vi "myBodePlot.vi"(3 "swp_data":dbl[][](array[numeric]), 4 "可用pico数":u16, 5 "幅值单位":u8(ring) items=["dB", "abs"], 8 "响应选项":u8=2, 9 "注入选项":u8=2, 11 "freqs, meas, coups":i32[][](array[numeric])) -> (0 "Pha":cluster{dbl[], dbl[]}[](graph), 1 "Mag":cluster{dbl[], dbl[]}[](graph))   [LabVIEW 2024]
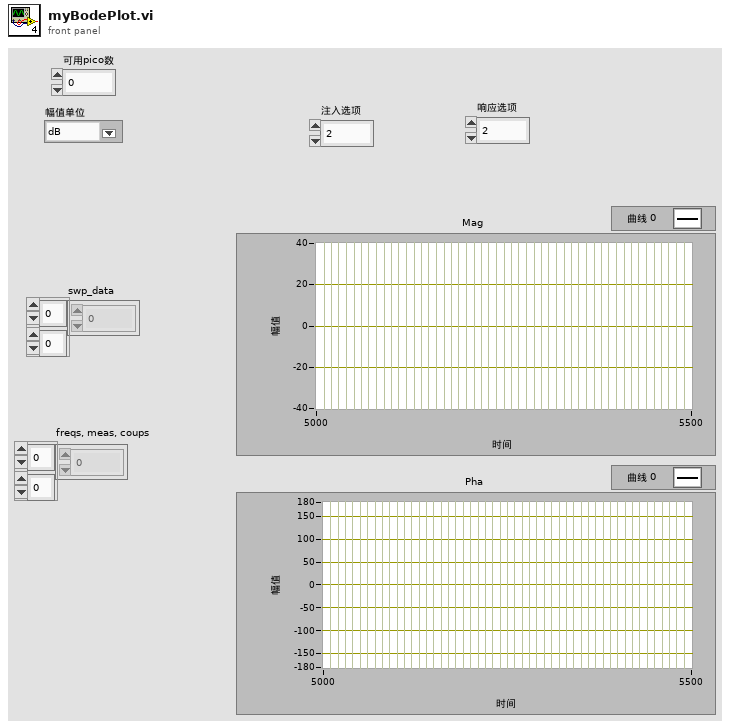
[diagram p1: front panel]
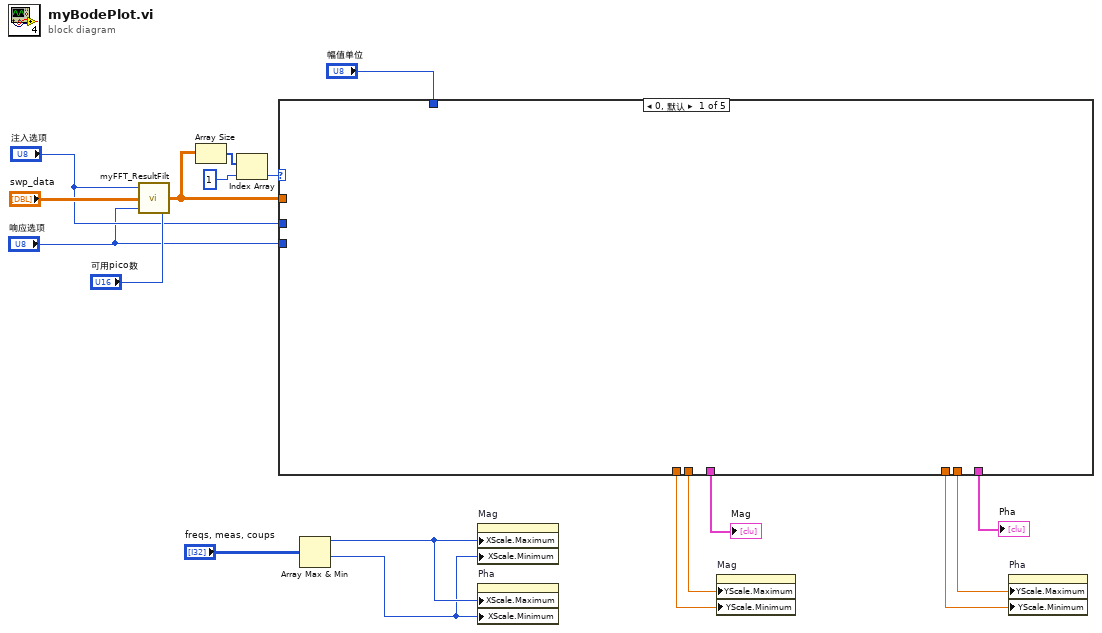
[diagram p0: block diagram]
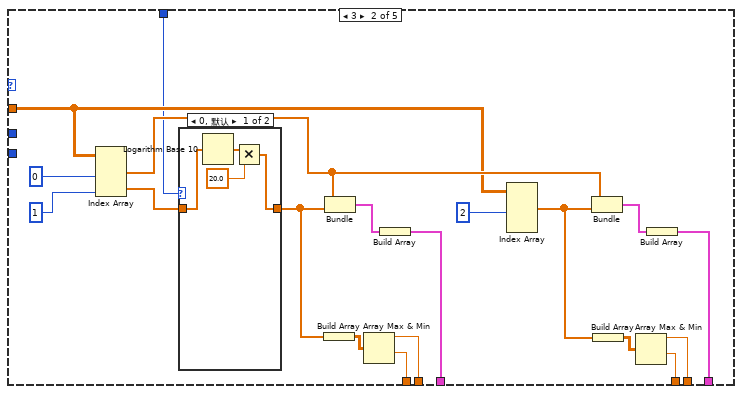
[diagram p2: hidden frame]
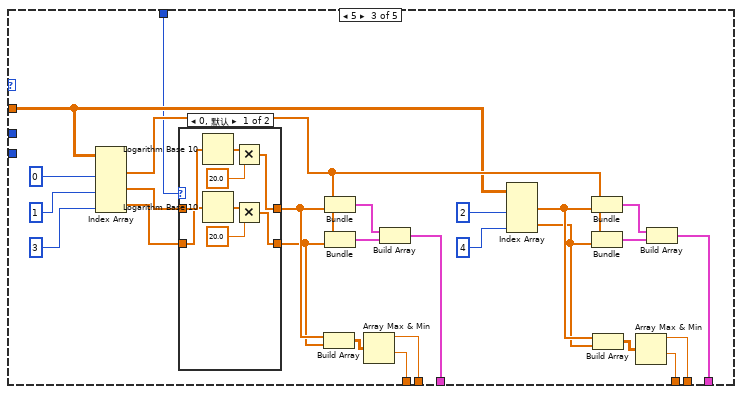
[diagram p4: hidden frame]
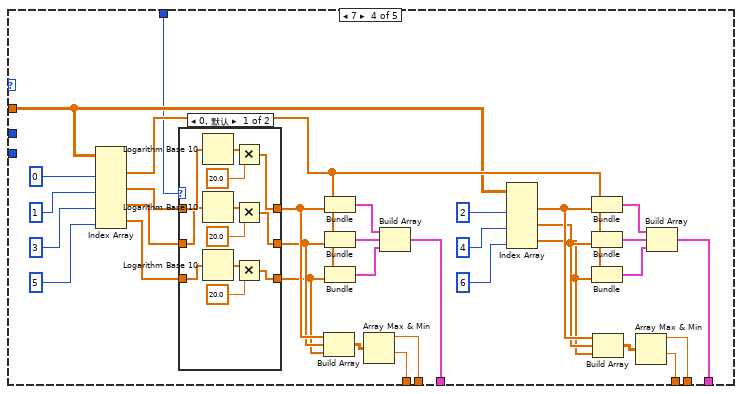
[diagram p6: hidden frame]
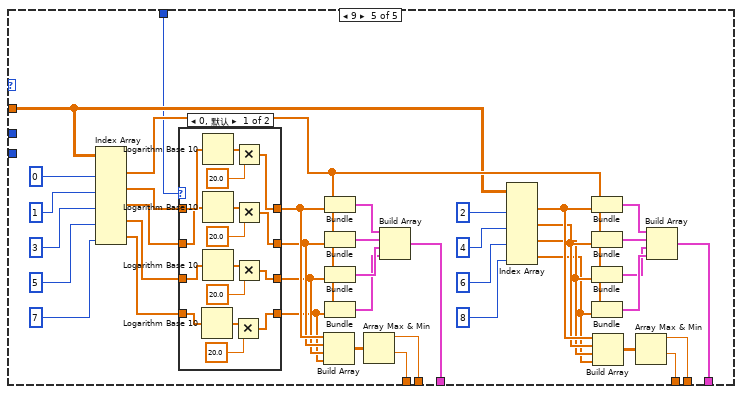
[diagram p8: hidden frame]
diagram:
  n1 = call "myFFT_ResultFilt.vi"("可用PICO数"="可用pico数", "响应选项"="响应选项", "写表结果输入"="swp_data", "注入选项"="注入选项") -> ("写表结果输出"=w2:dbl[][])  [unwired: 1 in]
  n2 = Array Size(array=w2) -> (size(s)=w13:i32[])
  n3 = Index Array(array=w13, index=1 ("索引")) -> (element=w11:i32)
  n4 = case shown="0, 默认" w11 {
    tunnel: "注入选项" -> [_ _ _ _ _]
    tunnel: "响应选项" -> [_ _ _ _ _]
    tunnel: "幅值单位" -> [_ w21 w49 w89 w141]
    tunnel: [_ w28 w56 w96 w148] -> w7
    tunnel: [_ w27 w55 w95 w147] -> w6
    tunnel: [_ w26 w54 w94 w146] -> w5
    tunnel: [_ w25 w53 w93 w145] -> w4
    tunnel: [_ w24 w52 w92 w144] -> w3
    tunnel: w2 -> [_ w23 w51 w91 w143]
    tunnel: [_ w22 w50 w90 w142] -> w1
    frame 0, Default {
    }
    frame 3 {
      n5 = Index Array(array=w23, index (col) #1=0, index (col) #2=1) -> (element #1=w29:dbl[], element #2=w19:dbl[])  [unwired: 2 in]
      n6 = case shown="0, 默认" w21 {
        tunnel: [w39 w42] -> w30
        tunnel: w19 -> [w38 w42]
        frame 0, Default {
          n7 = Logarithm Base 10(1:w38) -> (0:w41:dbl[])
          n8 = Multiply(x=w41, y=20.0) -> (x*y=w39:dbl[])
        }
        frame 1 {
        }
      }
      n9 = Build Array(w30) -> (w33:dbl[][])
      n10 = Bundle("写表结果输出"=w29, "写表结果输出"=w30) -> (w34:cluster{"写表结果输出":dbl[], "写表结果输出":dbl[]})  [unwired: 1 in]
      n11 = Array Max & Min(array=w33) -> (max value=w26:dbl, min value=w25:dbl)  [unwired: 2 out]
      n12 = Build Array(w34) -> (w22:cluster{"写表结果输出":dbl[], "写表结果输出":dbl[]}[])
      n13 = Index Array(array=w23, index (col) #1=2) -> (element #1=w32:dbl[])  [unwired: 3 in, 1 out]
      n14 = Bundle("写表结果输出"=w29, "写表结果输出"=w32) -> (w35:cluster{"写表结果输出":dbl[], "写表结果输出":dbl[]})  [unwired: 1 in]
      n15 = Build Array(w32) -> (w31:dbl[][])
      n16 = Array Max & Min(array=w31) -> (max value=w27:dbl, min value=w28:dbl)  [unwired: 2 out]
      n17 = Build Array(w35) -> (w24:cluster{"写表结果输出":dbl[], "写表结果输出":dbl[]}[])
    }
    frame 5 {
      n18 = Index Array(array=w51, index (col) #1=0, index (col) #2=1, index (col) #3=3) -> (element #1=w57:dbl[], element #2=w46:dbl[], element #3=w45:dbl[])  [unwired: 3 in]
      n19 = case shown="0, 默认" w49 {
        tunnel: [w74 w78] -> w59
        tunnel: w46 -> [w73 w78]
        tunnel: w45 -> [w70 w77]
        tunnel: [w69 w77] -> w58
        frame 0, Default {
          n20 = Logarithm Base 10(1:w73) -> (0:w76:dbl[])
          n21 = Logarithm Base 10(1:w70) -> (0:w71:dbl[])
          n22 = Multiply(x=w76, y=20.0) -> (x*y=w74:dbl[])
          n23 = Multiply(x=w71, y=20.0) -> (x*y=w69:dbl[])
        }
        frame 1 {
        }
      }
      n24 = Build Array(w59, w58) -> (w62:dbl[][])
      n25 = Bundle("写表结果输出"=w57, "写表结果输出"=w59) -> (w63:cluster{"写表结果输出":dbl[], "写表结果输出":dbl[]})  [unwired: 1 in]
      n26 = Bundle("写表结果输出"=w57, "写表结果输出"=w58) -> (w64:cluster{"写表结果输出":dbl[], "写表结果输出":dbl[]})  [unwired: 1 in]
      n27 = Array Max & Min(array=w62) -> (max value=w54:dbl, min value=w53:dbl)  [unwired: 2 out]
      n28 = Build Array(w63, w64) -> (w50:cluster{"写表结果输出":dbl[], "写表结果输出":dbl[]}[])
      n29 = Index Array(array=w51, index (col) #1=2, index (col) #2=4) -> (element #1=w61:dbl[], element #2=w44:dbl[])  [unwired: 2 in]
      n30 = Bundle("写表结果输出"=w57, "写表结果输出"=w61) -> (w66:cluster{"写表结果输出":dbl[], "写表结果输出":dbl[]})  [unwired: 1 in]
      n31 = Bundle("写表结果输出"=w57, "写表结果输出"=w44) -> (w65:cluster{"写表结果输出":dbl[], "写表结果输出":dbl[]})  [unwired: 1 in]
      n32 = Build Array(w61, w44) -> (w60:dbl[][])
      n33 = Array Max & Min(array=w60) -> (max value=w55:dbl, min value=w56:dbl)  [unwired: 2 out]
      n34 = Build Array(w66, w65) -> (w52:cluster{"写表结果输出":dbl[], "写表结果输出":dbl[]}[])
    }
    frame 7 {
      n35 = Index Array(array=w91, index (col) #1=0, index (col) #2=1, index (col) #3=3, index (col) #4=5) -> (element #1=w97:dbl[], element #2=w85:dbl[], element #3=w84:dbl[], element #4=w83:dbl[])  [unwired: 4 in]
      n36 = case shown="0, 默认" w89 {
        tunnel: [w121 w126] -> w100
        tunnel: w85 -> [w120 w126]
        tunnel: w84 -> [w115 w125]
        tunnel: w83 -> [w113 w124]
        tunnel: [w114 w125] -> w99
        tunnel: [w112 w124] -> w98
        frame 0, Default {
          n37 = Logarithm Base 10(1:w120) -> (0:w123:dbl[])
          n38 = Logarithm Base 10(1:w115) -> (0:w118:dbl[])
          n39 = Logarithm Base 10(1:w113) -> (0:w116:dbl[])
          n40 = Multiply(x=w123, y=20.0) -> (x*y=w121:dbl[])
          n41 = Multiply(x=w118, y=20.0) -> (x*y=w114:dbl[])
          n42 = Multiply(x=w116, y=20.0) -> (x*y=w112:dbl[])
        }
        frame 1 {
        }
      }
      n43 = Build Array(w100, w99, w98) -> (w103:dbl[][])
      n44 = Bundle("写表结果输出"=w97, "写表结果输出"=w100) -> (w104:cluster{"写表结果输出":dbl[], "写表结果输出":dbl[]})  [unwired: 1 in]
      n45 = Bundle("写表结果输出"=w97, "写表结果输出"=w99) -> (w105:cluster{"写表结果输出":dbl[], "写表结果输出":dbl[]})  [unwired: 1 in]
      n46 = Bundle("写表结果输出"=w97, "写表结果输出"=w98) -> (w106:cluster{"写表结果输出":dbl[], "写表结果输出":dbl[]})  [unwired: 1 in]
      n47 = Array Max & Min(array=w103) -> (max value=w94:dbl, min value=w93:dbl)  [unwired: 2 out]
      n48 = Build Array(w104, w105, w106) -> (w90:cluster{"写表结果输出":dbl[], "写表结果输出":dbl[]}[])
      n49 = Index Array(array=w91, index (col) #1=2, index (col) #2=4, index (col) #3=6) -> (element #1=w102:dbl[], element #2=w82:dbl[], element #3=w81:dbl[])  [unwired: 3 in]
      n50 = Bundle("写表结果输出"=w97, "写表结果输出"=w102) -> (w109:cluster{"写表结果输出":dbl[], "写表结果输出":dbl[]})  [unwired: 1 in]
      n51 = Bundle("写表结果输出"=w97, "写表结果输出"=w82) -> (w108:cluster{"写表结果输出":dbl[], "写表结果输出":dbl[]})  [unwired: 1 in]
      n52 = Bundle("写表结果输出"=w97, "写表结果输出"=w81) -> (w107:cluster{"写表结果输出":dbl[], "写表结果输出":dbl[]})  [unwired: 1 in]
      n53 = Build Array(w102, w82, w81) -> (w101:dbl[][])
      n54 = Array Max & Min(array=w101) -> (max value=w95:dbl, min value=w96:dbl)  [unwired: 2 out]
      n55 = Build Array(w109, w108, w107) -> (w92:cluster{"写表结果输出":dbl[], "写表结果输出":dbl[]}[])
    }
    frame 9 {
      n56 = Index Array(array=w143, index (col) #1=0, index (col) #2=1, index (col) #3=3, index (col) #4=5, index (col) #5=7) -> (element #1=w149:dbl[], element #2=w136:dbl[], element #3=w135:dbl[], element #4=w134:dbl[], element #5=w133:dbl[])  [unwired: 5 in]
      n57 = case shown="0, 默认" w141 {
        tunnel: [w180 w186] -> w153
        tunnel: w136 -> [w179 w186]
        tunnel: w135 -> [w174 w185]
        tunnel: w134 -> [w172 w184]
        tunnel: w133 -> [w168 w183]
        tunnel: [w173 w185] -> w152
        tunnel: [w171 w184] -> w151
        tunnel: [w167 w183] -> w150
        frame 0, Default {
          n58 = Logarithm Base 10(1:w168) -> (0:w170:dbl[])
          n59 = Logarithm Base 10(1:w179) -> (0:w182:dbl[])
          n60 = Logarithm Base 10(1:w174) -> (0:w177:dbl[])
          n61 = Logarithm Base 10(1:w172) -> (0:w175:dbl[])
          n62 = Multiply(x=w170, y=20.0) -> (x*y=w167:dbl[])
          n63 = Multiply(x=w182, y=20.0) -> (x*y=w180:dbl[])
          n64 = Multiply(x=w177, y=20.0) -> (x*y=w173:dbl[])
          n65 = Multiply(x=w175, y=20.0) -> (x*y=w171:dbl[])
        }
        frame 1 {
        }
      }
      n66 = Build Array(w153, w152, w151, w150) -> (w156:dbl[][])
      n67 = Bundle("写表结果输出"=w149, "写表结果输出"=w153) -> (w157:cluster{"写表结果输出":dbl[], "写表结果输出":dbl[]})  [unwired: 1 in]
      n68 = Bundle("写表结果输出"=w149, "写表结果输出"=w152) -> (w158:cluster{"写表结果输出":dbl[], "写表结果输出":dbl[]})  [unwired: 1 in]
      n69 = Bundle("写表结果输出"=w149, "写表结果输出"=w151) -> (w160:cluster{"写表结果输出":dbl[], "写表结果输出":dbl[]})  [unwired: 1 in]
      n70 = Bundle("写表结果输出"=w149, "写表结果输出"=w150) -> (w159:cluster{"写表结果输出":dbl[], "写表结果输出":dbl[]})  [unwired: 1 in]
      n71 = Array Max & Min(array=w156) -> (max value=w146:dbl, min value=w145:dbl)  [unwired: 2 out]
      n72 = Build Array(w157, w158, w160, w159) -> (w142:cluster{"写表结果输出":dbl[], "写表结果输出":dbl[]}[])
      n73 = Index Array(array=w143, index (col) #1=2, index (col) #2=4, index (col) #3=6, index (col) #4=8) -> (element #1=w155:dbl[], element #2=w132:dbl[], element #3=w131:dbl[], element #4=w127:dbl[])  [unwired: 4 in]
      n74 = Bundle("写表结果输出"=w149, "写表结果输出"=w155) -> (w164:cluster{"写表结果输出":dbl[], "写表结果输出":dbl[]})  [unwired: 1 in]
      n75 = Bundle("写表结果输出"=w149, "写表结果输出"=w132) -> (w163:cluster{"写表结果输出":dbl[], "写表结果输出":dbl[]})  [unwired: 1 in]
      n76 = Bundle("写表结果输出"=w149, "写表结果输出"=w131) -> (w161:cluster{"写表结果输出":dbl[], "写表结果输出":dbl[]})  [unwired: 1 in]
      n77 = Bundle("写表结果输出"=w149, "写表结果输出"=w127) -> (w162:cluster{"写表结果输出":dbl[], "写表结果输出":dbl[]})  [unwired: 1 in]
      n78 = Build Array(w155, w132, w131, w127) -> (w154:dbl[][])
      n79 = Array Max & Min(array=w154) -> (max value=w147:dbl, min value=w148:dbl)  [unwired: 2 out]
      n80 = Build Array(w164, w163, w161, w162) -> (w144:cluster{"写表结果输出":dbl[], "写表结果输出":dbl[]}[])
    }
  }
  "Mag" <- w1
  "Pha" <- w3
  n81 = Array Max & Min(array="freqs, meas, coups") -> (max value=w18:i32, min value=w17:i32)  [unwired: 2 out]
  n82 = property on="Mag" class="XYGraph (严格)"("XScale.Maximum"=w18, "XScale.Minimum"=w17) -> ()  [unwired: 2 in, 2 out]
  n83 = property on="Pha" class="XYGraph (严格)"("XScale.Maximum"=w18, "XScale.Minimum"=w17) -> ()  [unwired: 2 in, 2 out]
  n84 = property on="Mag" class="XYGraph (严格)"("YScale.Maximum"=w5, "YScale.Minimum"=w4) -> ()  [unwired: 2 in, 2 out]
  n85 = property on="Pha" class="XYGraph (严格)"("YScale.Maximum"=w6, "YScale.Minimum"=w7) -> ()  [unwired: 2 in, 2 out]
